vi "InfoTest.vi"(8 "error in":errorcluster, 10 "Seleziona Test":i32(ring) items=["Test Endurance"=36, "Test su Statore H100 dia 65"=31, "Test su Statore H100 dia 65"=29, "Test Endurance"=34, "Test su Statore H100 dia 65"=30, "Test su Statore H100 dia 65"=28, "Test su Statore H100 dia 65"=32, "Richiesta prova 1"=7, "Test Endurance"=35, "Richiesta prova 1"=5, "Richiesta prova 1"=6, "Test su Statore H100 dia 65"=27, "Test doppio carico per freni 50Nm/12rpm"=24], 11 "TestForBenchArray":T1[](array[typedef])) -> (0 "error out":errorcluster, 3 "Info Test":string)   [LabVIEW 2019]
doc: "Formatta le informazioni principali dei test in una info box più leggibile"
uses:
  ByteGSAPIBase/TypeDef/Test.ctl
  ByteGSAPIBase/TypeDef/Asset.ctl
  ByteGSAPIBase/ByteGSAPIBase.lvclass
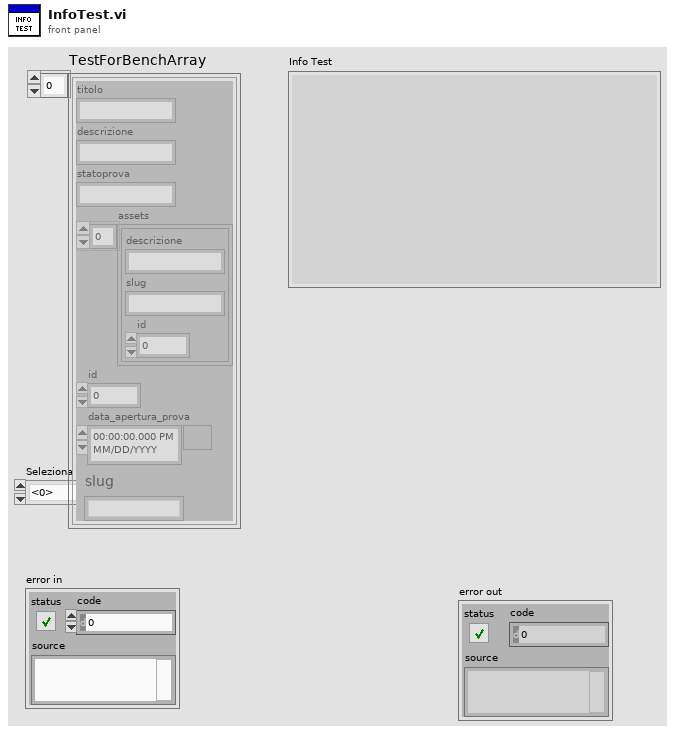
[diagram p1: front panel]
types:
  T1 = typedef "ByteGSWebAPI.lvlib/ByteGSAPIBase.lvclass/Test.ctl" = cluster{"titolo":string, "descrizione":string, "statoprova":string, "assets":T2[], "id":i32, "data_apertura_prova":timestamp, "slug":string}
  T2 = typedef "ByteGSWebAPI.lvlib/ByteGSAPIBase.lvclass/Asset.ctl" = cluster{"descrizione":string, "slug":string, "id":i32}
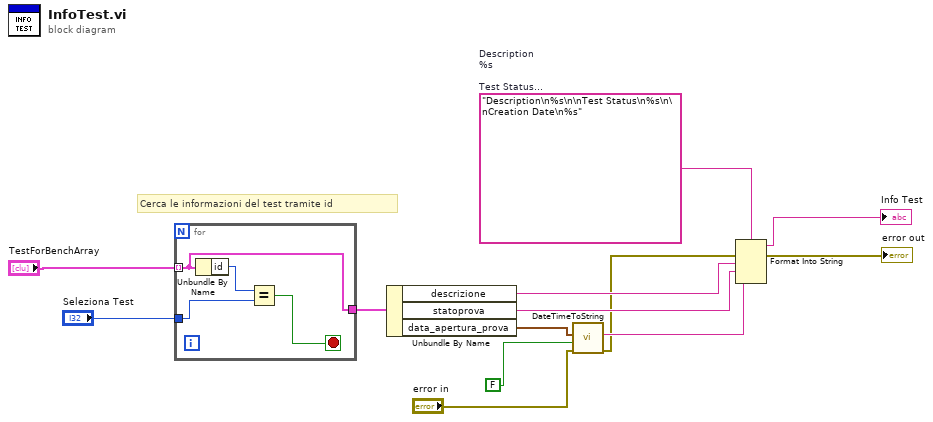
[diagram p0: block diagram]
diagram:
  w8 = "Description\n%s\n\nTest Status\n%s\n\nCreation Date\n%s"  # Description %s  Test Status %s  Creation Date %s
  # "Cerca le informazioni del test tramite id"
  n1 = for {
    tunnel: "TestForBenchArray" -> [w14] mode=indexing
    tunnel: "Seleziona Test" -> [w17]
    tunnel: [w14] -> w12
    stop <- w15 stop-if-true
    n2 = Unbundle By Name(w14) -> ("id"=w16:i32)
    n3 = Equal?(x=w16, y=w17) -> (x = y?=w15:bool)
  }
  n4 = Unbundle By Name(w12) -> ("descrizione"=w7:string, "statoprova"=w6:string, "data_apertura_prova"=w11:timestamp)
  n5 = call "DateTimeToString.vi"("error in"="error in", "current time"=w11, "include Time?"=FALSE ("Time")) -> ("error out"=w2:errorcluster, "date string"=w5:string)  [unwired: 7 in]
  n6 = Format Into String(format string=w8, error in=w2, w7, w6, w5) -> (resulting string=→"Info Test":string, error out=→"error out":errorcluster)  [unwired: 1 in]
